vi "VarArray_Replace elements.vi"(8 "Error In":errorcluster, 9 "Index Array In":i32[](array[numeric]), 10 "Replace Array In":variant[](array[variant]), 11 "Array In In In":variant[](array[variant])) -> (0 "Error Out":errorcluster, 1 "Replaced Indexs Out":i32[](array[numeric]), 2 "Replaced Data Out":variant[](array[variant]), 3 "Array Out":variant[](array[variant]))   [LabVIEW 2015]
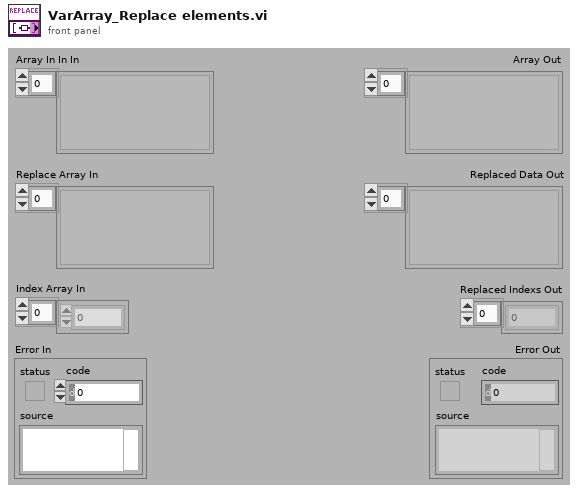
[diagram p1: front panel]
types:
  T1 = enum16{"Size to Primary", "Size to Secondary", "Size to Largest", "Size to Smallest"}
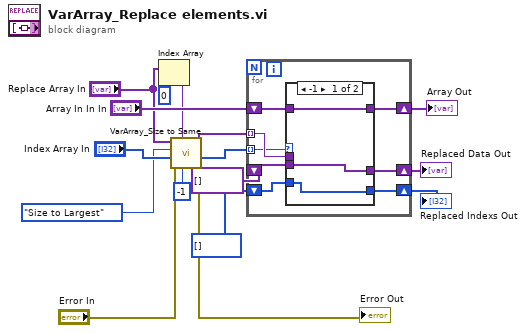
[diagram p0: block diagram]
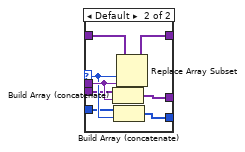
[diagram p2: hidden frame]
diagram:
  n1 = Index Array(array="Replace Array In", index=0) -> (element=w6:variant)
  n2 = call "VarArray_Size to Same.vi"("Secondary Default In"=-1 ("Secondary default"), "Primary Default In"=w6, "Error In"="Error In", "Secondary Array In"="Index Array In", "Select In"=T1."Size to Largest" ("select"), "Primary Array In"="Replace Array In") -> ("Error Out"=→"Error Out":errorcluster, "Secondary Array Out"=w14:i32[], "Primary Array Out"=w10:variant[])  [unwired: 3 in]
  n3 = for {
    tunnel: w14 -> [w21] mode=indexing
    tunnel: w10 -> [w22] mode=indexing
    shift-right: [w23] -> w16
    shift-left: "Array In In In" -> [w24]
    shift-right: [w20] -> w4
    shift-left: variant[] [] -> [w18]
    shift-right: [w19] -> w3
    shift-left: i32[] [] -> [w17]
    n4 = case shown="-1" w21 {
      selector: w21 -> [_ w32]
      tunnel: w24 -> [w27 w35]
      tunnel: [w27 w34] -> w23
      tunnel: w22 -> [_ w33]
      tunnel: [w25 w31] -> w20
      tunnel: [w26 w29] -> w19
      tunnel: w18 -> [w25 w30]
      tunnel: w17 -> [w26 w28]
      frame -1 {
      }
      frame Default {
        n5 = Build Array (concatenate)(w30, w33) -> (w31:variant[])
        n6 = Build Array (concatenate)(w28, w32) -> (w29:i32[])
        n7 = Replace Array Subset(array=w35, new element=w33, index=w32) -> (w34:variant[])
      }
    }
  }
  "Array Out" <- w16
  "Replaced Data Out" <- w4
  "Replaced Indexs Out" <- w3
